vi "GUI - System Parameters.vi"(10 "Caller VI FilePath":path) -> ()   [LabVIEW 2014]
uses:
  Custom Controls/TypeDef - System Configuration.ctl
  FileIO/TypeDef - File Actions.ctl
panel:
  in  "Apply":bool
  in  "HW Configuration (each Station)":T1={"Results FilePath"=path "", "Analysis Parameters"={"Area"={"Lower Value"=50000.0, "Upper Value"=150000.0}, "Circle Filter Radius"={"Lower Value"=50.0, "Upper Value"=500.0}, "Edge Detection Threshold"=50}, "ROI Parameters"={"ROI size (in Radius)"={"Width"=1.0, "Height"=0.5}}}
  in  "Return":bool
  # "Units\nArea = [pixel-squared]\nCircle Radius = [pixel]\nEdge Detection Threshold=Intensity Difference\n              theoretically, 0-65535. Realistically 0-2048\nROI width and Height = Radius multiplier, \n        so absolute size may change based on size of egg sac"
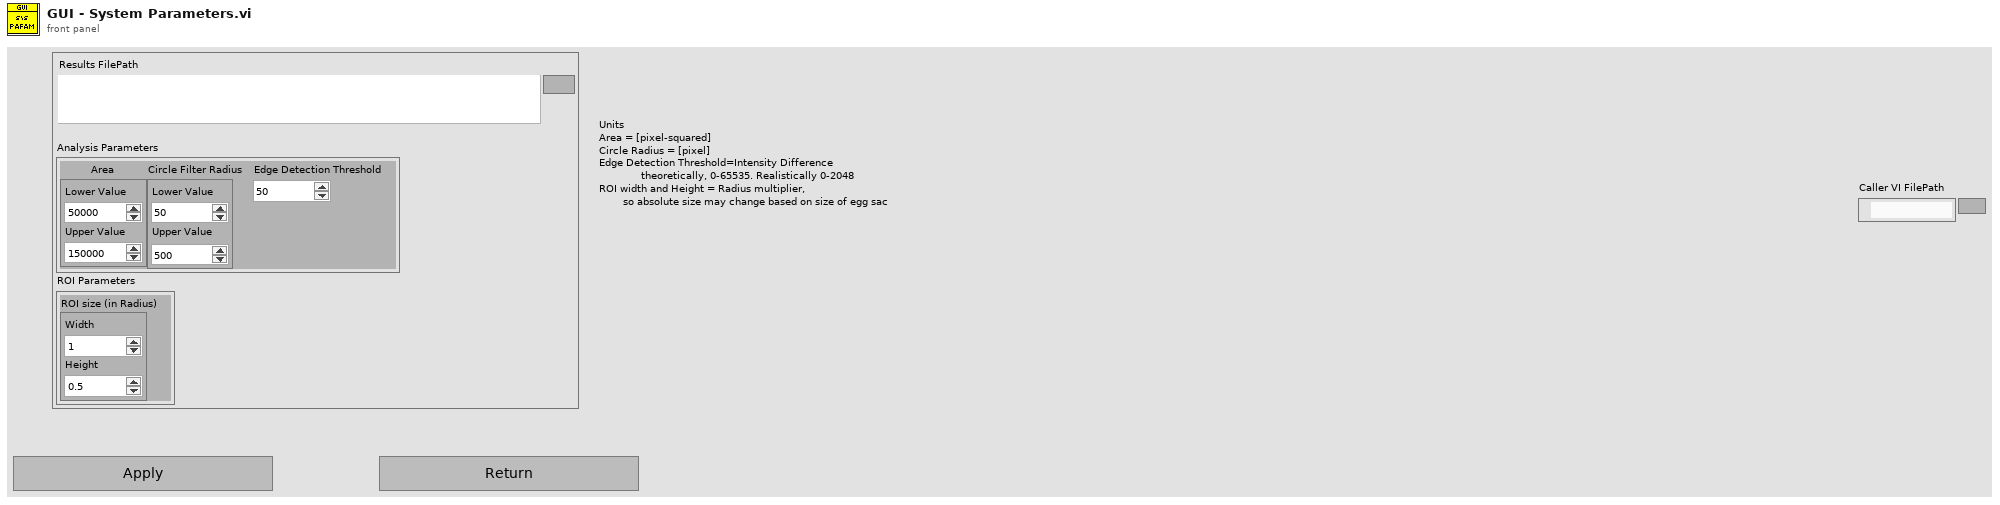
[diagram p1: front panel]
types:
  T1 = typedef "TypeDef - System Configuration.ctl" = cluster{"Results FilePath":path, "Analysis Parameters":cluster{"Area":cluster{"Lower Value":dbl, "Upper Value":dbl}, "Circle Filter Radius":cluster{"Lower Value":sgl, "Upper Value":sgl}, "Edge Detection Threshold":u16}, "ROI Parameters":cluster{"ROI size (in Radius)":cluster{"Width":dbl, "Height":dbl}}}
  T2 = typedef "TypeDef - File Actions.ctl" = enum16{"Read", "Write", "Get Current"}
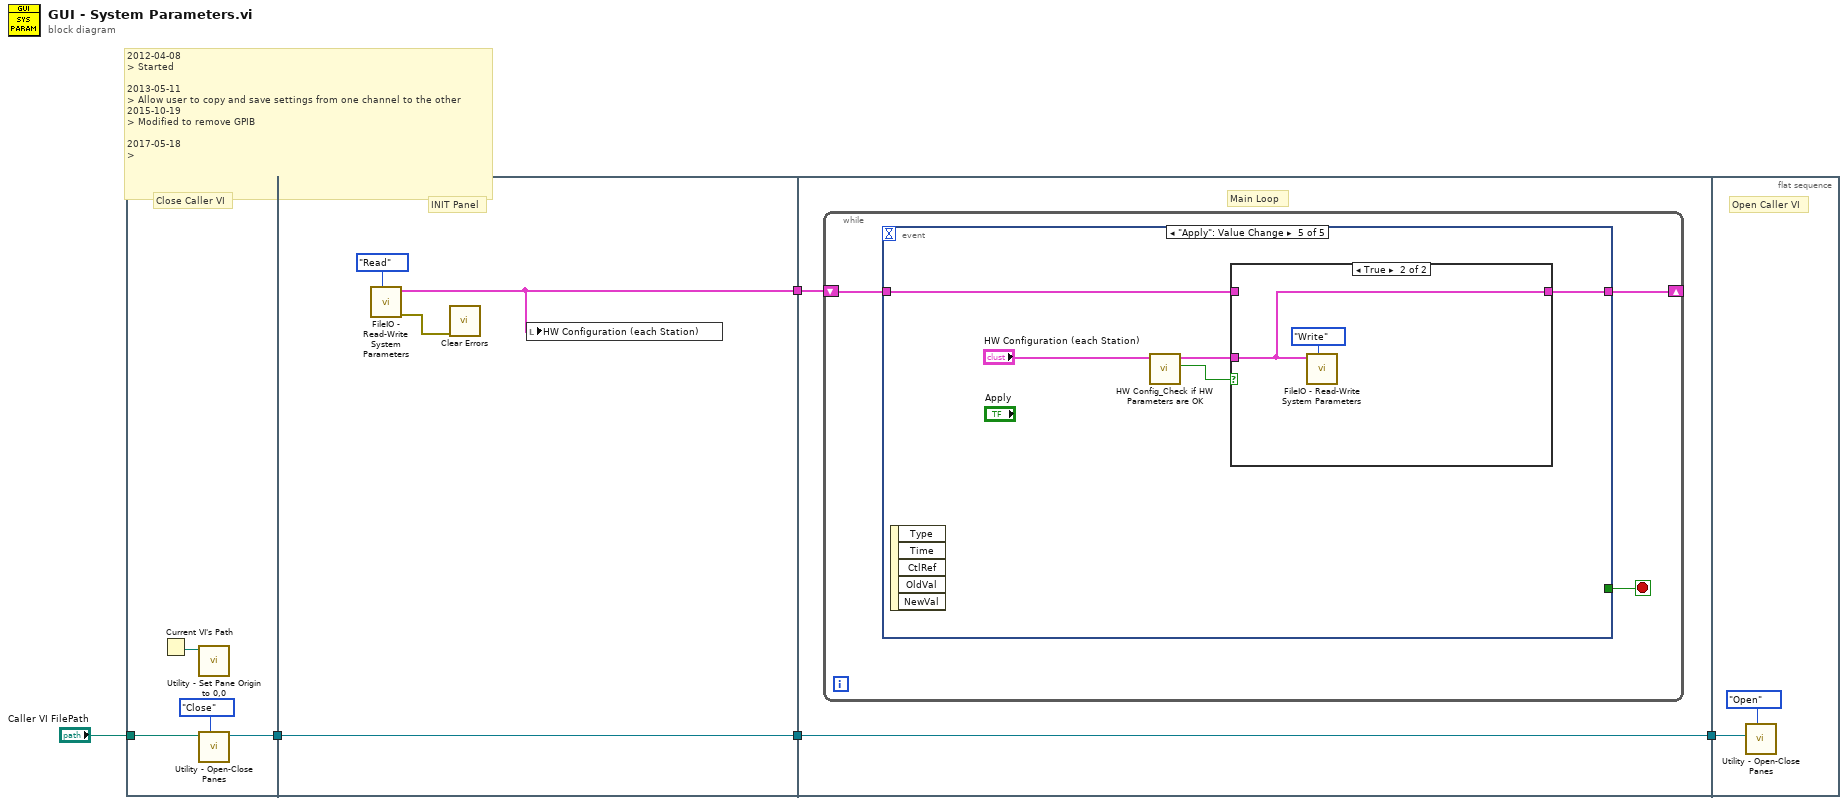
[diagram p0: block diagram]
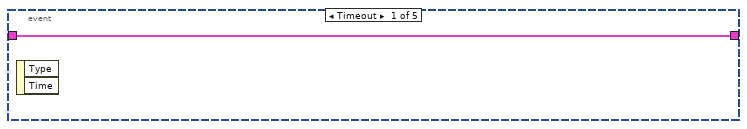
[diagram p2: hidden frame]
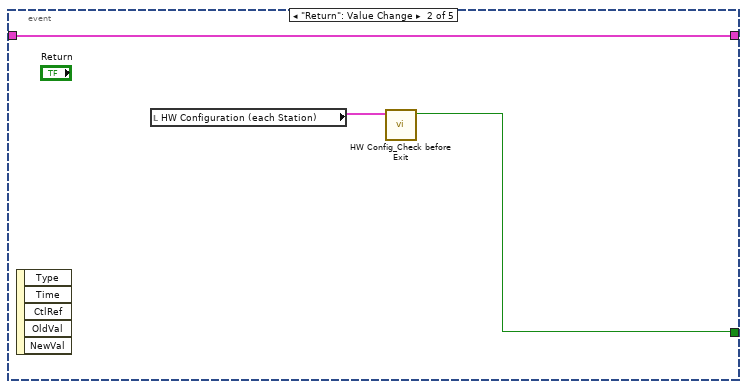
[diagram p3: hidden frame]
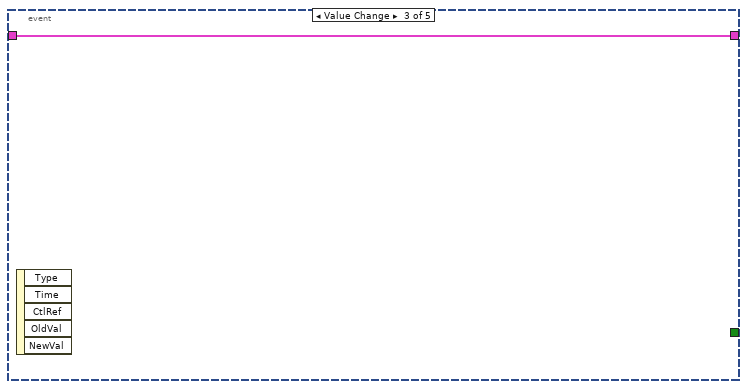
[diagram p4: hidden frame]
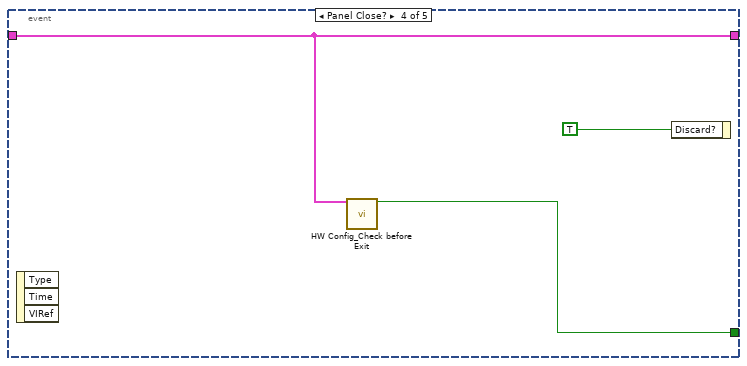
[diagram p5: hidden frame]
diagram:
  # "2012-04-08\n> Started\n\n2013-05-11\n> Allow user to copy and save settings from one channel to the other\n2015-10-19\n> Modified to remove GPIB\n\n2017-05-18\n>"
  n1 = flat-sequence {
    tunnel: [w8] -> w4
    tunnel: "Caller VI FilePath" -> [w7]
    tunnel: w4 -> [w13]
    tunnel: [w13] -> w3
    tunnel: [w11] -> w1
    tunnel: [w15] -> w2
    tunnel: w3 -> [w15]
    tunnel: w1 -> [w14]
    tunnel: w2 -> [w35]
    frame #0 {
      # "Close Caller VI"
      n2 = Current VI's Path() -> (path=w6:path)
      n3 = call "Utility - Set Pane Origin to 0,0.vi"("vi path"=w6) -> ()  [unwired: 10 in, 1 out]
      n4 = call "Utility - Open-Close Panes.vi"("Panel Type"=enum16{"Open", "Close"}."Close", "FilePath"=w7) -> ("VI Reference Out"=w8:refnum<vi>)  [unwired: 8 in, 1 out]
    }
    frame #1 {
      # "INIT Panel"
      n5 = call "FileIO - Read-Write System Parameters.vi"("Action"=TypeDef_-_File_Actions."Read") -> ("error out"=w10:errorcluster, "System Parameters out"=w11:T1)  [unwired: 9 in]
      n6 = call <vilib>:"Clear Errors.vi"("error in (no error)"=w10) -> ()  [unwired: 5 in, 2 out]
      n7 = local write "HW Configuration (each Station)"(w11) -> ()
    }
    frame #2 {
      # "Main Loop"
      n8 = while {
        shift-right: [w17] -> _
        shift-left: w14 -> [w16]
        stop <- w18 stop-if-true
        n9 = event shown="[4] \"Apply\": Value Change" {
          selector: _ -> [_ _ _ _ _]
          dyn-events: _ -> [_ _ _ _ _]
          timeout: _ -> [_ _ _ _ _]
          tunnel: [_ w21 _ w26 _] -> w18
          tunnel: [w19 w22 w23 w25 w30] -> w17
          tunnel: w16 -> [w19 w22 w23 w25 w28]
          event Timeout {
            n10 = event-data() -> ()  [unwired: 1 in, 2 out]
          }
          event "Return": Value Change {
            n11 = event-data() -> ()  [unwired: 1 in, 5 out]
            n12 = local read "HW Configuration (each Station)"() -> (w20:T1)
            n13 = call "HW Config_Check before Exit.vi"("HW Configuration (each Station)"=w20) -> ("T button?"=w21:bool)  [unwired: 10 in]
          }
          event Value Change {
            n14 = event-data() -> ()  [unwired: 1 in, 5 out]
          }
          event Panel Close? {
            n15 = event-data() -> ()  [unwired: 1 in, 3 out]
            n16 = call "HW Config_Check before Exit.vi"("HW Configuration (each Station)"=w25) -> ("T button?"=w26:bool)  [unwired: 10 in]
            n17 = event-data("Discard?"=TRUE) -> ()  [unwired: 1 in, 1 out]
          }
          event "Apply": Value Change {
            n18 = event-data() -> ()  [unwired: 1 in, 5 out]
            n19 = call "HW Config_Check if HW Parameters are OK.vi"("HW Configuration (each Station)"="HW Configuration (each Station)") -> ("Info OK?"=w31:bool, "HW Configuration (each Station)"=w29:T1)  [unwired: 9 in]
            n20 = case shown="True" w31 {
              tunnel: w29 -> [_ w33]
              tunnel: [w32 w33] -> w30
              tunnel: w28 -> [w32 _]
              frame False {
              }
              frame True {
                n21 = call "FileIO - Read-Write System Parameters.vi"("Action"=TypeDef_-_File_Actions."Write", "System Parameters in"=w33) -> ()  [unwired: 8 in, 2 out]
              }
            }
          }
        }
      }
    }
    frame #3 {
      # "Open Caller VI"
      n22 = call "Utility - Open-Close Panes.vi"("Panel Type"=enum16{"Open", "Close"}."Open", "VI Reference In"=w35) -> ()  [unwired: 8 in, 2 out]
    }
  }
